vi "Update Point Data.vi"(9 "Data":variant, 10 "Point Ident":string, 11 "ITask Actor in":refnum<class "ITask Actor.lvclass">) -> (3 "ITask Actor out":refnum<class "ITask Actor.lvclass">)   [LabVIEW 2023, in "ITask Actor.lvlib" / "ITask Actor.lvclass"]
uses:
  ITask Actor.lvclass
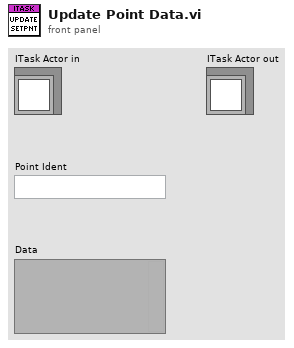
[diagram p1: front panel]
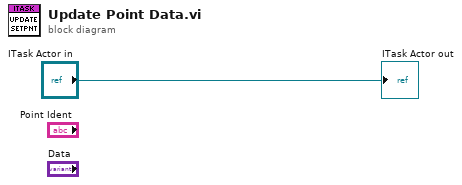
[diagram p0: block diagram]
diagram:
  "ITask Actor out" <- "ITask Actor in"
